vi "SendTcpPlacedCommand.vi"(6 "機器番号":u8, 10 "Sample Name":string="Sample", 11 "アドレス":string) -> (1 "送信文字列":string, 2 "空?":bool, 3 "Send List Out":cluster{"Address":string, "Data":string}[](array[cluster]))   [LabVIEW 2017]
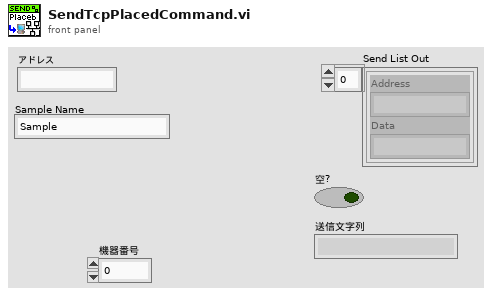
[diagram p1: front panel]
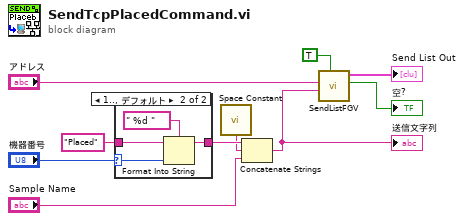
[diagram p0: block diagram]
diagram:
  n1 = case shown="1.., デフォルト" "機器番号" {
    selector: "機器番号" -> [_ w13]
    tunnel: [w11 w15] -> w4
    tunnel: "Placed" ("要素") -> [w11 w12]
    frame 0 {
    }
    frame 1.., Default {
      n2 = Format Into String(format string=" %d " ("形式文字列"), initial string=w12, w13) -> (resulting string=w15:string)  [unwired: 1 in, 1 out]
    }
  }
  n3 = call <vilib>:"Space Constant.vi"() -> ("String"=w1:string)
  n4 = Concatenate Strings(w4, w1, "Sample Name") -> (w3:string)
  "送信文字列" <- w3
  n5 = call "SendListFGV.vi"("Set"=TRUE, "Data"=w3, "アドレス"="アドレス") -> ("空?"=→"空?":bool, "Send List Out"=→"Send List Out":cluster{"Address":string, "Data":string}[])  [unwired: 6 in, 1 out]
